vi "App - analyze RUS V6.vi"() -> ()   [LabVIEW 2015] (continued)
"z (pi/2)"=0.44352845258494766+0.2180214777125745i, "z center"=0.028000000000000025+0.0040000000000000036i, "z(0)"=-0.18602147771257446+0.41952845258494764i, "radius"=0.4674067691314655}}, "timestamp(min)"=396.73333333432674, "timestamp"=timestamp(3493751625 s since 1904-01-01), "Magn Field(T)"=0.0}, {"temperature"=137.004, "lorentzian"={"Amplitude"=0.00024818777938784227, "omega(0)"=668.2077960895239, "Gamma"=0.053536500417424936, "phase"=3.575640217162926, "Q"=12481.349936575929, "Norm  Ampl"=0.024927732275848467, "z (inf)"=0.22381537528742693-0.41844465648109325i, "4corners"={"z (-pi/2)"=-0.3944446564810932-0.1918153752874269i, "z(inf)"=0.22381537528742693-0.41844465648109325i, "z (pi/2)"=0.4504446564810933+0.1998153752874269i, "z center"=0.028000000000000025+0.0040000000000000036i, "z(0)"=-0.16781537528742688+0.42644465648109325i, "radius"=0.46562125057645803}}, "timestamp(min)"=398.0666666701436, "timestamp"=timestamp(3493751705 s since 1904-01-01), "Magn Field(T)"=0.0}, {"temperature"=136.689, "lorentzian"={"Amplitude"=0.0002522590875798226, "omega(0)"=668.216668111389, "Gamma"=0.053803366985016095, "phase"=3.6082228025377545, "Q"=12419.606904851944, "Norm  Ampl"=0.02511881590690244, "z (inf)"=0.23803210631804037-0.4129506304339384i, "4corners"={"z (-pi/2)"=-0.3889506304339384-0.20603210631804034i, "z(inf)"=0.23803210631804037-0.4129506304339384i, "z (pi/2)"=0.44495063043393845+0.21403210631804034i, "z center"=0.028000000000000025+0.0040000000000000036i, "z(0)"=-0.18203210631804032+0.42095063043393843i, "radius"=0.46686327110156284}}, "timestamp(min)"=399.3833333328366, "timestamp"=timestamp(3493751784 s since 1904-01-01), "Magn Field(T)"=0.0}, {"temperature"=136.379, "lorentzian"={"Amplitude"=0.0002437959945548481, "omega(0)"=668.2220891882298, "Gamma"=0.052047760738563105, "phase"=3.5758353326684773, "Q"=12838.632819281545, "Norm  Ampl"=0.0242465841922333, "z (inf)"=0.22399512738349894-0.4186163112320136i, "4corners"={"z (-pi/2)"=-0.3946163112320136-0.19199512738349891i, "z(inf)"=0.22399512738349894-0.4186163112320136i, "z (pi/2)"=0.4506163112320136+0.19999512738349892i, "z center"=0.028000000000000025+0.0040000000000000036i, "z(0)"=-0.1679951273834989+0.4266163112320136i, "radius"=0.4658525909313247}}, "timestamp(min)"=400.7166666686535, "timestamp"=timestamp(3493751864 s since 1904-01-01), "Magn Field(T)"=0.0}, {"temperature"=136.08, "lorentzian"={"Amplitude"=0.00024364628649236486, "omega(0)"=668.2279899714331, "Gamma"=0.05257683433154817, "phase"=3.562128551223608, "Q"=12709.551620350601, "Norm  Ampl"=0.02452040469231934, "z (inf)"=0.2183965576468025-0.4217378607902434i, "4corners"={"z (-pi/2)"=-0.39773786079024337-0.18639655764680246i, "z(inf)"=0.2183965576468025-0.4217378607902434i, "z (pi/2)"=0.4537378607902434+0.19439655764680247i, "z center"=0.028000000000000025+0.0040000000000000036i, "z(0)"=-0.16239655764680244+0.4297378607902434i, "radius"=0.4663727857347648}}, "timestamp(min)"=402.0333333313465, "timestamp"=timestamp(3493751943 s since 1904-01-01), "Magn Field(T)"=0.0}, {"temperature"=135.77, "lorentzian"={"Amplitude"=0.00022800803606069718, "omega(0)"=668.2341074013727, "Gamma"=0.049576251679184384, "phase"=3.5174097869555605, "Q"=13478.91550425432, "Norm  Ampl"=0.023118481798097362, "z (inf)"=0.19915533730309165-0.42977618112069815i, "4corners"={"z (-pi/2)"=-0.40577618112069813-0.16715533730309162i, "z(inf)"=0.19915533730309165-0.42977618112069815i, "z (pi/2)"=0.4617761811206982+0.17515533730309163i, "z center"=0.028000000000000025+0.0040000000000000036i, "z(0)"=-0.1431553373030916+0.43777618112069816i, "radius"=0.4663216966805124}}, "timestamp(min)"=403.3500000014901, "timestamp"=timestamp(3493752022 s since 1904-01-01), "Magn Field(T)"=0.0}, {"temperature"=135.475, "lorentzian"={"Amplitude"=0.00021967242445661102, "omega(0)"=668.2403250081744, "Gamma"=0.048208626694876563, "phase"=3.5063922887652854, "Q"=13861.426280354768, "Norm  Ampl"=0.02254989139105604, "z (inf)"=0.19487774885740458-0.43297576868681537i, "4corners"={"z (-pi/2)"=-0.40897576868681534-0.16287774885740455i, "z(inf)"=0.19487774885740458-0.43297576868681537i, "z (pi/2)"=0.4649757686868154+0.17087774885740456i, "z center"=0.028000000000000025+0.0040000000000000036i, "z(0)"=-0.13887774885740453+0.4409757686868154i, "radius"=0.4677563526913858}}, "timestamp(min)"=404.683333337307, "timestamp"=timestamp(3493752102 s since 1904-01-01), "Magn Field(T)"=0.0}, {"temperature"=135.167, "lorentzian"={"Amplitude"=0.00022045956380851477, "omega(0)"=668.2467222103966, "Gamma"=0.04866848493880481, "phase"=3.5042890577355816, "Q"=13730.584032986486, "Norm  Ampl"=0.022778847947626805, "z (inf)"=0.19405932289046807-0.4335919440676238i, "4corners"={"z (-pi/2)"=-0.4095919440676238-0.16205932289046804i, "z(inf)"=0.19405932289046807-0.4335919440676238i, "z (pi/2)"=0.46559194406762383+0.17005932289046805i, "z center"=0.028000000000000025+0.0040000000000000036i, "z(0)"=-0.13805932289046802+0.4415919440676238i, "radius"=0.4680410326368011}}, "timestamp(min)"=406.0, "timestamp"=timestamp(3493752181 s since 1904-01-01), "Magn Field(T)"=0.0}, {"temperature"=134.859, "lorentzian"={"Amplitude"=0.00020373450011305496, "omega(0)"=668.2497252249998, "Gamma"=0.04534069328819745, "phase"=3.4590588773416715, "Q"=14738.409952786287, "Norm  Ampl"=0.021363968760541766, "z (inf)"=0.1750860858123121-0.4436420009483996i, "4corners"={"z (-pi/2)"=-0.4196420009483996-0.14308608581231208i, "z(inf)"=0.1750860858123121-0.4436420009483996i, "z (pi/2)"=0.47564200094839965+0.1510860858123121i, "z center"=0.028000000000000025+0.0040000000000000036i, "z(0)"=-0.11908608581231206+0.4516420009483996i, "radius"=0.471187518566307}}, "timestamp(min)"=407.3166666701436, "timestamp"=timestamp(3493752260 s since 1904-01-01), "Magn Field(T)"=0.0}, {"temperature"=134.565, "lorentzian"={"Amplitude"=0.00022308585172458564, "omega(0)"=668.2550593154574, "Gamma"=0.04913914581717594, "phase"=3.50838853037322, "Q"=13599.240446745365, "Norm  Ampl"=0.02307832843849415, "z (inf)"=0.20442977527987274-0.43441189720743484i, "4corners"={"z (-pi/2)"=-0.4024118972074348-0.1644297752798727i, "z(inf)"=0.20442977527987274-0.43441189720743484i, "z (pi/2)"=0.4744118972074349+0.17242977527987272i, "z center"=0.03600000000000003+0.0040000000000000036i, "z(0)"=-0.13242977527987268+0.44241189720743485i, "radius"=0.46965261716916984}}, "timestamp(min)"=408.6499999985099, "timestamp"=timestamp(3493752340 s since 1904-01-01), "Magn Field(T)"=0.0}, {"temperature"=134.259, "lorentzian"={"Amplitude"=0.000209359984950497, "omega(0)"=668.2609151074342, "Gamma"=0.04650212304347896, "phase"=3.5133547690153906, "Q"=14370.546361563273, "Norm  Ampl"=0.02182407268942164, "z (inf)"=0.19848174926920006-0.4332540514538913i, "4corners"={"z (-pi/2)"=-0.40925405145389127-0.16648174926920004i, "z(inf)"=0.19848174926920006-0.4332540514538913i, "z (pi/2)"=0.4652540514538913+0.17448174926920004i, "z center"=0.028000000000000025+0.0040000000000000036i, "z(0)"=-0.14248174926920001+0.4412540514538913i, "radius"=0.4693134691725016}}, "timestamp(min)"=409.9666666686535, "timestamp"=timestamp(3493752419 s since 1904-01-01), "Magn Field(T)"=0.0}, {"temperature"=133.967, "lorentzian"={"Amplitude"=0.00016795569051138588, "omega(0)"=668.2619254491482, "Gamma"=0.04198266024418475, "phase"=3.3789707396391027, "Q"=15917.56981483118, "Norm  Ampl"=0.017415878698290484, "z (inf)"=0.14155055450548604-0.31120218603325117i, "4corners"={"z (-pi/2)"=-0.3592021860332511-0.005550554505486041i, "z(inf)"=0.14155055450548604-0.31120218603325117i, "z (pi/2)"=0.4472021860332512+0.18955055450548597i, "z center"=0.04400000000000004+0.09199999999999997i, "z(0)"=-0.05355055450548597+0.4952021860332511i, "radius"=0.4148350437298183}}, "timestamp(min)"=411.30000000447035, "timestamp"=timestamp(3493752499 s since 1904-01-01), "Magn Field(T)"=0.0}, {"temperature"=133.655, "lorentzian"={"Amplitude"=0.00020618932515028255, "omega(0)"=668.270115071191, "Gamma"=0.046136883483514225, "phase"=3.5346323148739778, "Q"=14484.509238903822, "Norm  Ampl"=0.021552558999279797, "z (inf)"=0.20691517073138083-0.42752368430412885i, "4corners"={"z (-pi/2)"=-0.4035236843041288-0.1749151707313808i, "z(inf)"=0.20691517073138083-0.42752368430412885i, "z (pi/2)"=0.4595236843041289+0.1829151707313808i, "z center"=0.028000000000000025+0.0040000000000000036i, "z(0)"=-0.15091517073138078+0.43552368430412886i, "radius"=0.4671437984531622}}, "timestamp(min)"=412.6166666671634, "timestamp"=timestamp(3493752578 s since 1904-01-01), "Magn Field(T)"=0.0}, {"temperature"=133.359, "lorentzian"={"Amplitude"=0.00019301381489978157, "omega(0)"=668.276245083583, "Gamma"=0.04348621694234654, "phase"=3.531368153146456, "Q"=15367.5415355071, "Norm  Ampl"=0.02015177614748303, "z (inf)"=0.20408538557141195-0.4246479987406104i, "4corners"={"z (-pi/2)"=-0.40064799874061036-0.17208538557141193i, "z(inf)"=0.20408538557141195-0.4246479987406104i, "z (pi/2)"=0.4566479987406104+0.18008538557141193i, "z center"=0.028000000000000025+0.0040000000000000036i, "z(0)"=-0.1480853855714119+0.4326479987406104i, "radius"=0.4634060528695791}}, "timestamp(min)"=413.933333337307, "timestamp"=timestamp(3493752657 s since 1904-01-01), "Magn Field(T)"=0.0}, {"temperature"=133.076, "lorentzian"={"Amplitude"=0.00019974392460320753, "omega(0)"=668.2795802722522, "Gamma"=0.04461745326656678, "phase"=3.53671447289831, "Q"=14977.985773406179, "Norm  Ampl"=0.020699137011803485, "z (inf)"=0.21457417147702626-0.4241791203195198i, "4corners"={"z (-pi/2)"=-0.3921791203195198-0.17457417147702622i, "z(inf)"=0.21457417147702626-0.4241791203195198i, "z (pi/2)"=0.46417912031951986+0.18257417147702623i, "z center"=0.03600000000000003+0.0040000000000000036i, "z(0)"=-0.1425741714770262+0.4321791203195198i, "radius"=0.46392466392325404}}, "timestamp(min)"=415.26666666567326, "timestamp"=timestamp(3493752737 s since 1904-01-01), "Magn Field(T)"=0.0}, {"temperature"=132.767, "lorentzian"={"Amplitude"=0.00020954228159723317, "omega(0)"=668.2870233031718, "Gamma"=0.046821008502632336, "phase"=3.6004118876433644, "Q"=14273.230002416542, "Norm  Ampl"=0.021889480609721925, "z (inf)"=0.24305720211583082-0.41516193523764255i, "4corners"={"z (-pi/2)"=-0.3831619352376425-0.20305720211583078i, "z(inf)"=0.24305720211583082-0.41516193523764255i, "z (pi/2)"=0.4551619352376426+0.2110572021158308i, "z center"=0.03600000000000003+0.0040000000000000036i, "z(0)"=-0.17105720211583075+0.42316193523764256i, "radius"=0.46751407775616943}}, "timestamp(min)"=416.58333333581686, "timestamp"=timestamp(3493752816 s since 1904-01-01), "Magn Field(T)"=0.0}, {"temperature"=132.465, "lorentzian"={"Amplitude"=0.00019413049707023668, "omega(0)"=668.2869168107318, "Gamma"=0.04319877501840161, "phase"=3.55325340676782, "Q"=15470.043225208541, "Norm  Ampl"=0.020176299526293698, "z (inf)"=0.2148844854302435-0.42403811821360354i, "4corners"={"z (-pi/2)"=-0.4000381182136035-0.18288448543024347i, "z(inf)"=0.2148844854302435-0.42403811821360354i, "z (pi/2)"=0.45603811821360357+0.19088448543024347i, "z center"=0.028000000000000025+0.0040000000000000036i, "z(0)"=-0.15888448543024344+0.43203811821360355i, "radius"=0.46705721441636006}}, "timestamp(min)"=417.91666666418314, "timestamp"=timestamp(3493752896 s since 1904-01-01), "Magn Field(T)"=0.0}, {"temperature"=132.185, "lorentzian"={"Amplitude"=0.00020122225797151018, "omega(0)"=668.2934784041765, "Gamma"=0.04497947268960905, "phase"=3.5446976448663943, "Q"=14857.74373158809, "Norm  Ampl"=0.020912876525446128, "z (inf)"=0.21038601556727435-0.4316763214619255i, "4corners"={"z (-pi/2)"=-0.3996763214619255-0.18638601556727433i, "z(inf)"=0.21038601556727435-0.4316763214619255i, "z (pi/2)"=0.45567632146192555+0.17838601556727432i, "z center"=0.028000000000000025-0.0040000000000000036i, "z(0)"=-0.1543860155672743+0.4236763214619255i, "radius"=0.4649426788473073}}, "timestamp(min)"=419.23333333432674, "timestamp"=timestamp(3493752975 s since 1904-01-01), "Magn Field(T)"=0.0}, {"temperature"=131.882, "lorentzian"={"Amplitude"=0.00017903490059702695, "omega(0)"=668.3008315870534, "Gamma"=0.04055671373632796, "phase"=3.5607932411011722, "Q"=16478.180059949846, "Norm  Ampl"=0.018542520405159534, "z (inf)"=0.21409420197942536-0.41361295774797074i, "4corners"={"z (-pi/2)"=-0.3896129577479707-0.18209420197942533i, "z(inf)"=0.21409420197942536-0.41361295774797074i, "z (pi/2)"=0.4456129577479708+0.19009420197942534i, "z center"=0.028000000000000025+0.0040000000000000036i, "z(0)"=-0.1580942019794253+0.42161295774797075i, "radius"=0.45719977525078415}}, "timestamp(min)"=420.55000000447035, "timestamp"=timestamp(3493753054 s since 1904-01-01), "Magn Field(T)"=0.0}, {"temperature"=131.592, "lorentzian"={"Amplitude"=0.00017776941850395074, "omega(0)"=668.3028814309054, "Gamma"=0.040071528004769166, "phase"=3.556601894504015, "Q"=16677.748883231165, "Norm  Ampl"=0.018550360511525102, "z (inf)"=0.21465311273870263-0.419634170792521i, "4corners"={"z (-pi/2)"=-0.395634170792521-0.1826531127387026i, "z(inf)"=0.21465311273870263-0.419634170792521i, "z (pi/2)"=0.45163417079252105+0.1906531127387026i, "z center"=0.028000000000000025+0.0040000000000000036i, "z(0)"=-0.15865311273870258+0.42763417079252103i, "radius"=0.4629311991625902}}, "timestamp(min)"=421.8833333328366, "timestamp"=timestamp(3493753134 s since 1904-01-01), "Magn Field(T)"=0.0}, {"temperature"=131.299, "lorentzian"={"Amplitude"=0.00013151959831981622, "omega(0)"=668.3062964998082, "Gamma"=0.03348268101980571, "phase"=3.467971571661652, "Q"=19959.760573070325, "Norm  Ampl"=0.01370925850354954, "z (inf)"=0.17527374281445499-0.29582856805960495i, "4corners"={"z (-pi/2)"=-0.3438285680596049-0.039273742814454976i, "z(inf)"=0.17527374281445499-0.29582856805960495i, "z (pi/2)"=0.43182856805960496+0.22327374281445492i, "z center"=0.04400000000000004+0.09199999999999997i, "z(0)"=-0.08727374281445491+0.4798285680596049i, "radius"=0.40944327293982896}}, "timestamp(min)"=423.20000000298023, "timestamp"=timestamp(3493753213 s since 1904-01-01), "Magn Field(T)"=0.0}, {"temperature"=131.007, "lorentzian"={"Amplitude"=0.00014024604190308675, "omega(0)"=668.3103990781085, "Gamma"=0.0354379197218754, "phase"=3.487085072823789, "Q"=18858.623878691407, "Norm  Ampl"=0.014555488747515302, "z (inf)"=0.183098526053321-0.29446138419265844i, "4corners"={"z (-pi/2)"=-0.34246138419265837-0.04709852605332099i, "z(inf)"=0.183098526053321-0.29446138419265844i, "z (pi/2)"=0.43046138419265845+0.23109852605332093i, "z center"=0.04400000000000004+0.09199999999999997i, "z(0)"=-0.09509852605332092+0.4784613841926584i, "radius"=0.4107320311618171}}, "timestamp(min)"=424.51666666567326, "timestamp"=timestamp(3493753292 s since 1904-01-01), "Magn Field(T)"=0.0}, {"temperature"=130.718, "lorentzian"={"Amplitude"=0.00018728871691243128, "omega(0)"=668.310674127471, "Gamma"=0.04173713236217242, "phase"=3.4962997673810627, "Q"=16012.37642126991, "Norm  Ampl"=0.019142027382721867, "z (inf)"=0.18729046326062257-0.43408232050414974i, "4corners"={"z (-pi/2)"=-0.4020823205041497-0.16329046326062255i, "z(inf)"=0.18729046326062257-0.43408232050414974i, "z (pi/2)"=0.45808232050414976+0.15529046326062254i, "z center"=0.028000000000000025-0.0040000000000000036i, "z(0)"=-0.13129046326062252+0.42608232050414974i, "radius"=0.4586330276986361}}, "timestamp(min)"=425.8500000014901, "timestamp"=timestamp(3493753372 s since 1904-01-01), "Magn Field(T)"=0.0}, {"temperature"=130.427, "lorentzian"={"Amplitude"=0.00013102976571802591, "omega(0)"=668.3160212015783, "Gamma"=0.03289666447607903, "phase"=3.479634497746158, "Q"=20315.616547919246, "Norm  Ampl"=0.013442055183748003, "z (inf)"=0.18751308439089182-0.293489351771138i, "4corners"={"z (-pi/2)"=-0.3334893517711379-0.0435130843908918i, "z(inf)"=0.18751308439089182-0.293489351771138i, "z (pi/2)"=0.437489351771138+0.22751308439089174i, "z center"=0.052000000000000046+0.09199999999999997i, "z(0)"=-0.08351308439089172+0.47748935177113794i, "radius"=0.40861453274457227}}, "timestamp(min)"=427.16666666418314, "timestamp"=timestamp(3493753451 s since 1904-01-01), "Magn Field(T)"=0.0}, {"temperature"=130.147, "lorentzian"={"Amplitude"=0.00019806996039286532, "omega(0)"=668.3205621538442, "Gamma"=0.04395504205226639, "phase"=3.5868870379071494, "Q"=15204.639353072454, "Norm  Ampl"=0.02022729371515346, "z (inf)"=0.22621098732741798-0.4193063264724261i, "4corners"={"z (-pi/2)"=-0.3873063264724261-0.20221098732741796i, "z(inf)"=0.22621098732741798-0.4193063264724261i, "z (pi/2)"=0.4433063264724261+0.19421098732741796i, "z center"=0.028000000000000025-0.0040000000000000036i, "z(0)"=-0.17021098732741793+0.4113063264724261i, "radius"=0.46018142107796056}}, "timestamp(min)"=428.5, "timestamp"=timestamp(3493753531 s since 1904-01-01), "Magn Field(T)"=0.0}, {"temperature"=129.849, "lorentzian"={"Amplitude"=0.00018012359308280804, "omega(0)"=668.3261810591241, "Gamma"=0.03572807603918743, "phase"=3.617601804019526, "Q"=18705.910173447, "Norm  Ampl"=0.01846804924972829, "z (inf)"=0.17686465617028402-0.4314417557280484i, "4corners"={"z (-pi/2)"=-0.5194417557280484-0.208864656170284i, "z(inf)"=0.17686465617028402-0.4314417557280484i, "z (pi/2)"=0.3994417557280484+0.26486465617028404i, "z center"=-0.06+0.028000000000000025i, "z(0)"=-0.296864656170284+0.48744175572804843i, "radius"=0.5169057866276393}}, "timestamp(min)"=429.8166666701436, "timestamp"=timestamp(3493753610 s since 1904-01-01), "Magn Field(T)"=0.0}, {"temperature"=129.561, "lorentzian"={"Amplitude"=0.0002515206474333576, "omega(0)"=668.3339307703254, "Gamma"=0.05293578222265151, "phase"=3.697878467065015, "Q"=12625.371775168398, "Norm  Ampl"=0.026109156013374792, "z (inf)"=0.24843944779595978-0.5028560864052527i, "4corners"={"z (-pi/2)"=-0.43085608640525264-0.3444394477959598i, "z(inf)"=0.24843944779595978-0.5028560864052527i, "z (pi/2)"=0.4068560864052526+0.17643944779595977i, "z center"=-0.01200000000000001-0.08400000000000002i, "z(0)"=-0.2724394477959598+0.3348560864052526i, "radius"=0.4932232020971732}}, "timestamp(min)"=431.1333333328366, "timestamp"=timestamp(3493753689 s since 1904-01-01), "Magn Field(T)"=0.0}, {"temperature"=129.282, "lorentzian"={"Amplitude"=0.00019009529834722127, "omega(0)"=668.3324079597492, "Gamma"=0.042712971939908764, "phase"=3.5856365991332066, "Q"=15647.059373438127, "Norm  Ampl"=0.019869211365660003, "z (inf)"=0.2278387908458529-0.42406748951978035i, "4corners"={"z (-pi/2)"=-0.3920674895197803-0.20383879084585288i, "z(inf)"=0.2278387908458529-0.42406748951978035i, "z (pi/2)"=0.44806748951978037+0.19583879084585287i, "z center"=0.028000000000000025-0.0040000000000000036i, "z(0)"=-0.17183879084585285+0.41606748951978034i, "radius"=0.465179791132615}}, "timestamp(min)"=432.4666666686535, "timestamp"=timestamp(3493753769 s since 1904-01-01), "Magn Field(T)"=0.0}, {"temperature"=128.991, "lorentzian"={"Amplitude"=0.00020743270166107407, "omega(0)"=668.3322615543187, "Gamma"=0.04692462104458906, "phase"=3.5328468712785126, "Q"=14242.677866684338, "Norm  Ampl"=0.021731792084702495, "z (inf)"=0.2046104571630927-0.4321239265355797i, "4corners"={"z (-pi/2)"=-0.40012392653557965-0.18061045716309268i, "z(inf)"=0.2046104571630927-0.4321239265355797i, "z (pi/2)"=0.4561239265355797+0.17261045716309267i, "z center"=0.028000000000000025-0.0040000000000000036i, "z(0)"=-0.14861045716309265+0.4241239265355797i, "radius"=0.4631213124566813}}, "timestamp(min)"=433.7833333313465, "timestamp"=timestamp(3493753848 s since 1904-01-01), "Magn Field(T)"=0.0}, {"temperature"=128.717, "lorentzian"={"Amplitude"=0.00014057972242425618, "omega(0)"=668.3288000801537, "Gamma"=0.0350239817019726, "phase"=3.350369108098308, "Q"=19082.03372669397, "Norm  Ampl"=0.014440672605235712, "z (inf)"=0.12945625364420338-0.3113549647555858i, "4corners"={"z (-pi/2)"=-0.3593549647555857+0.006543746355796645i, "z(inf)"=0.12945625364420338-0.3113549647555858i, "z (pi/2)"=0.4473549647555858+0.1774562536442033i, "z center"=0.04400000000000004+0.09199999999999997i, "z(0)"=-0.041456253644203286+0.4953549647555857i, "radius"=0.41230813584003195}}, "timestamp(min)"=435.1000000014901, "timestamp"=timestamp(3493753927 s since 1904-01-01), "Magn Field(T)"=0.0}, {"temperature"=128.421, "lorentzian"={"Amplitude"=0.00018912094504794594, "omega(0)"=668.3337947654519, "Gamma"=0.0420370819340677, "phase"=3.45940499769483, "Q"=15898.672410556183, "Norm  Ampl"=0.019525044126968823, "z (inf)"=0.18114246269768364-0.44521177378260157i, "4corners"={"z (-pi/2)"=-0.40521177378260154-0.1491424626976836i, "z(inf)"=0.18114246269768364-0.44521177378260157i, "z (pi/2)"=0.4772117737826016+0.1411424626976836i, "z center"=0.03600000000000003-0.0040000000000000036i, "z(0)"=-0.10914246269768357+0.43721177378260156i, "radius"=0.46447191928289705}}, "timestamp(min)"=436.433333337307, "timestamp"=timestamp(3493754007 s since 1904-01-01), "Magn Field(T)"=0.0}, {"temperature"=128.135, "lorentzian"={"Amplitude"=0.0001945195497852276, "omega(0)"=668.3393724178951, "Gamma"=0.043849594993256275, "phase"=3.4896884528609635, "Q"=15241.631593648253, "Norm  Ampl"=0.020523623085199085, "z (inf)"=0.18765440283338847-0.44397435687764764i, "4corners"={"z (-pi/2)"=-0.4119743568776476-0.16365440283338845i, "z(inf)"=0.18765440283338847-0.44397435687764764i, "z (pi/2)"=0.46797435687764766+0.15565440283338844i, "z center"=0.028000000000000025-0.0040000000000000036i, "z(0)"=-0.13165440283338842+0.43597435687764763i, "radius"=0.46804589844798933}}, "timestamp(min)"=437.75, "timestamp"=timestamp(3493754086 s since 1904-01-01), "Magn Field(T)"=0.0}, {"temperature"=127.874, "lorentzian"={"Amplitude"=0.000190466492974867, "omega(0)"=668.3408415336296, "Gamma"=0.04304683332538277, "phase"=3.5244127391147786, "Q"=15525.900278930372, "Norm  Ampl"=0.02009953162829439, "z (inf)"=0.2104132227577419-0.43712420258490553i, "4corners"={"z (-pi/2)"=-0.3971242025849055-0.17841322275774188i, "z(inf)"=0.2104132227577419-0.43712420258490553i, "z (pi/2)"=0.46912420258490556+0.17041322275774187i, "z center"=0.03600000000000003-0.0040000000000000036i, "z(0)"=-0.13841322275774184+0.4291242025849055i, "radius"=0.4669224208983244}}, "timestamp(min)"=439.08333333581686, "timestamp"=timestamp(3493754166 s since 1904-01-01), "Magn Field(T)"=0.0}, {"temperature"=127.58, "lorentzian"={"Amplitude"=0.00017614434719281864, "omega(0)"=668.3350781624661, "Gamma"=0.03977774583620109, "phase"=3.4103259526571854, "Q"=16801.733333873963, "Norm  Ampl"=0.018474740713941437, "z (inf)"=0.15131608902790966-0.45177914883439746i, "4corners"={"z (-pi/2)"=-0.41977914883439743-0.12731608902790964i, "z(inf)"=0.15131608902790966-0.45177914883439746i, "z (pi/2)"=0.4757791488343975+0.11931608902790963i, "z center"=0.028000000000000025-0.0040000000000000036i, "z(0)"=-0.09531608902790961+0.44377914883439745i, "radius"=0.4644491618508928}}, "timestamp(min)"=440.3999999985099, "timestamp"=timestamp(3493754245 s since 1904-01-01), "Magn Field(T)"=0.0}, {"temperature"=127.303, "lorentzian"={"Amplitude"=0.000178448287164071, "omega(0)"=668.341978511539, "Gamma"=0.04075165439042157, "phase"=3.458727986906405, "Q"=16400.36431670928, "Norm  Ampl"=0.018933127124076275, "z (inf)"=0.18088296555633987-0.44542949587281366i, "4corners"={"z (-pi/2)"=-0.40542949587281363-0.14888296555633984i, "z(inf)"=0.18088296555633987-0.44542949587281366i, "z (pi/2)"=0.4774294958728137+0.14088296555633983i, "z center"=0.03600000000000003-0.0040000000000000036i, "z(0)"=-0.1088829655563398+0.43742949587281366i, "radius"=0.4645977545521781}}, "timestamp(min)"=441.7166666686535, "timestamp"=timestamp(3493754324 s since 1904-01-01), "Magn Field(T)"=0.0}, {"temperature"=127.032, "lorentzian"={"Amplitude"=0.0001793737910586766, "omega(0)"=668.3443633787955, "Gamma"=0.04031506960918336, "phase"=3.482825666306089, "Q"=16578.028262328822, "Norm  Ampl"=0.018801002983454388, "z (inf)"=0.19206426889851805-0.43546318642137727i, "4corners"={"z (-pi/2)"=-0.40346318642137724-0.152064268898518i, "z(inf)"=0.19206426889851805-0.43546318642137727i, "z (pi/2)"=0.4754631864213773+0.16006426889851802i, "z center"=0.03600000000000003+0.0040000000000000036i, "z(0)"=-0.12006426889851798+0.4434631864213773i, "radius"=0.46635174305073546}}, "timestamp(min)"=443.05000000447035, "timestamp"=timestamp(3493754404 s since 1904-01-01), "Magn Field(T)"=0.0}, {"temperature"=126.745, "lorentzian"={"Amplitude"=0.00017473128234191018, "omega(0)"=668.3397547361191, "Gamma"=0.03922736347643625, "phase"=3.4158312259381005, "Q"=17037.59048546784, "Norm  Ampl"=0.018213770062324868, "z (inf)"=0.16174244705836888-0.45096228744718125i, "4corners"={"z (-pi/2)"=-0.4109622874471812-0.12974244705836885i, "z(inf)"=0.16174244705836888-0.45096228744718125i, "z (pi/2)"=0.4829622874471813+0.12174244705836884i, "z center"=0.03600000000000003-0.0040000000000000036i, "z(0)"=-0.08974244705836881+0.44296228744718125i, "radius"=0.46431287877060157}}, "timestamp(min)"=444.3666666671634, "timestamp"=timestamp(3493754483 s since 1904-01-01), "Magn Field(T)"=0.0}, {"temperature"=126.472, "lorentzian"={"Amplitude"=0.00016985229184637778, "omega(0)"=668.338634717693, "Gamma"=0.038548010622264324, "phase"=3.36580870245142, "Q"=17337.824285325845, "Norm  Ampl"=0.017944948936428617, "z (inf)"=0.1395051514979586-0.4578694336986776i, "4corners"={"z (-pi/2)"=-0.4178694336986776-0.1075051514979586i, "z(inf)"=0.1395051514979586-0.4578694336986776i, "z (pi/2)"=0.48986943369867764+0.09950515149795859i, "z center"=0.03600000000000003-0.0040000000000000036i, "z(0)"=-0.06750515149795856+0.4498694336986776i, "radius"=0.46552205021091503}}, "timestamp(min)"=445.70000000298023, "timestamp"=timestamp(3493754563 s since 1904-01-01), "Magn Field(T)"=0.0}, {"temperature"=126.195, "lorentzian"={"Amplitude"=0.0001697476143014984, "omega(0)"=668.3411059711797, "Gamma"=0.0389192723855822, "phase"=3.400885738644188, "Q"=17172.49745446858, "Norm  Ampl"=0.0181237265906366, "z (inf)"=0.15539779092559663-0.45410803111628234i, "4corners"={"z (-pi/2)"=-0.4141080311162823-0.12339779092559659i, "z(inf)"=0.15539779092559663-0.45410803111628234i, "z (pi/2)"=0.48610803111628237+0.11539779092559659i, "z center"=0.03600000000000003-0.0040000000000000036i, "z(0)"=-0.08339779092559656+0.44610803111628233i, "radius"=0.46567485669003933}}, "timestamp(min)"=447.01666666567326, "timestamp"=timestamp(3493754642 s since 1904-01-01), "Magn Field(T)"=0.0}, {"temperature"=125.926, "lorentzian"={"Amplitude"=0.00014967332960728232, "omega(0)"=668.3387712789065, "Gamma"=0.03405009771839295, "phase"=3.343347027084076, "Q"=19628.10141710365, "Norm  Ampl"=0.015778792659266735, "z (inf)"=0.1288598639328376-0.4579999888655082i, "4corners"={"z (-pi/2)"=-0.41799998886550815-0.09685986393283756i, "z(inf)"=0.1288598639328376-0.4579999888655082i, "z (pi/2)"=0.4899999888655082+0.08885986393283755i, "z center"=0.03600000000000003-0.0040000000000000036i, "z(0)"=-0.056859863932837526+0.4499999888655082i, "radius"=0.4633993355837993}}, "timestamp(min)"=448.33333333581686, "timestamp"=timestamp(3493754721 s since 1904-01-01), "Magn Field(T)"=0.0}, {"temperature"=125.648, "lorentzian"={"Amplitude"=0.00015890027273297025, "omega(0)"=668.3427557708224, "Gamma"=0.03654471251520353, "phase"=3.4071524057178104, "Q"=18288.35718690562, "Norm  Ampl"=0.017102639047579412, "z (inf)"=0.15882428088801925-0.45558704635195746i, "4corners"={"z (-pi/2)"=-0.4155870463519574-0.12682428088801923i, "z(inf)"=0.15882428088801925-0.45558704635195746i, "z (pi/2)"=0.4875870463519575+0.1188242808880192i, "z center"=0.03600000000000003-0.0040000000000000036i, "z(0)"=-0.08682428088801918+0.44758704635195745i, "radius"=0.46799216276401895}}, "timestamp(min)"=449.66666666418314, "timestamp"=timestamp(3493754801 s since 1904-01-01), "Magn Field(T)"=0.0}, {"temperature"=125.371, "lorentzian"={"Amplitude"=0.00014113258135423898, "omega(0)"=668.3438270287197, "Gamma"=0.0328359775535354, "phase"=3.4224417889228933, "Q"=20354.010351574263, "Norm  Ampl"=0.015317995908975795, "z (inf)"=0.16530066288420467-0.4442230921647853i, "4corners"={"z (-pi/2)"=-0.41222309216478525-0.12530066288420463i, "z(inf)"=0.16530066288420467-0.4442230921647853i, "z (pi/2)"=0.4842230921647853+0.13330066288420464i, "z center"=0.03600000000000003+0.0040000000000000036i, "z(0)"=-0.0933006628842046+0.4522230921647853i, "radius"=0.4665003770331342}}, "timestamp(min)"=450.98333333432674, "timestamp"=timestamp(3493754880 s since 1904-01-01), "Magn Field(T)"=0.0}, {"temperature"=125.102, "lorentzian"={"Amplitude"=0.0001429072723984059, "omega(0)"=668.3463481103089, "Gamma"=0.03319261106950844, "phase"=3.4922376591079947, "Q"=20135.395396003318, "Norm  Ampl"=0.015660205089643275, "z (inf)"=0.19806430364890984-0.439089658276503i, "4corners"={"z (-pi/2)"=-0.40708965827650295-0.1580643036489098i, "z(inf)"=0.19806430364890984-0.439089658276503i, "z (pi/2)"=0.479089658276503+0.1660643036489098i, "z center"=0.03600000000000003+0.0040000000000000036i, "z(0)"=-0.12606430364890978+0.447089658276503i, "radius"=0.47179792685936445}}, "timestamp(min)"=452.30000000447035, "timestamp"=timestamp(3493754959 s since 1904-01-01), "Magn Field(T)"=0.0}, {"temperature"=124.83, "lorentzian"={"Amplitude"=0.00013813052592595213, "omega(0)"=668.3455084349229, "Gamma"=0.03220463241618305, "phase"=3.4504535565686507, "Q"=20753.08607152661, "Norm  Ampl"=0.015278154630597103, "z (inf)"=0.18020770874129619-0.4479597969299136i, "4corners"={"z (-pi/2)"=-0.4159597969299136-0.14020770874129615i, "z(inf)"=0.18020770874129619-0.4479597969299136i, "z (pi/2)"=0.48795979692991365+0.14820770874129616i, "z center"=0.03600000000000003+0.0040000000000000036i, "z(0)"=-0.10820770874129612+0.4559597969299136i, "radius"=0.474408601630855}}, "timestamp(min)"=453.6333333328366, "timestamp"=timestamp(3493755039 s since 1904-01-01), "Magn Field(T)"=0.0}, {"temperature"=124.565, "lorentzian"={"Amplitude"=0.0001241550689128081, "omega(0)"=668.3450708618282, "Gamma"=0.029302305447045547, "phase"=3.3705378321996333, "Q"=22808.61729701255, "Norm  Ampl"=0.013845225294181049, "z (inf)"=0.1432331585027775-0.4561669504399603i, "4corners"={"z (-pi/2)"=-0.4241669504399603-0.10323315850277746i, "z(inf)"=0.1432331585027775-0.4561669504399603i, "z (pi/2)"=0.49616695043996034+0.11123315850277747i, "z center"=0.03600000000000003+0.0040000000000000036i, "z(0)"=-0.07123315850277744+0.4641669504399603i, "radius"=0.47249610851275237}}, "timestamp(min)"=454.95000000298023, "timestamp"=timestamp(3493755118 s since 1904-01-01), "Magn Field(T)"=0.0}, {"temperature"=124.29, "lorentzian"={"Amplitude"=0.00013600574422085066, "omega(0)"=668.3433267141062, "Gamma"=0.03222809761528601, "phase"=3.303602764581753, "Q"=20737.90810404851, "Norm  Ampl"=0.015235315667254033, "z (inf)"=0.11225308169717747-0.4625435119875039i, "4corners"={"z (-pi/2)"=-0.43054351198750385-0.07225308169717744i, "z(inf)"=0.11225308169717747-0.4625435119875039i, "z (pi/2)"=0.5025435119875039+0.08025308169717744i, "z center"=0.03600000000000003+0.0040000000000000036i, "z(0)"=-0.04025308169717741+0.4705435119875039i, "radius"=0.4727339431920989}}, "timestamp(min)"=456.2833333313465, "timestamp"=timestamp(3493755198 s since 1904-01-01), "Magn Field(T)"=0.0}, {"temperature"=124.019, "lorentzian"={"Amplitude"=0.00011823441411221721, "omega(0)"=668.3444873126522, "Gamma"=0.027985877204057336, "phase"=3.332408594972943, "Q"=23881.491455117117, "Norm  Ampl"=0.013390117286503522, "z (inf)"=0.13474472920756247-0.46577566662945014i, "4corners"={"z (-pi/2)"=-0.4257756666294501-0.08674472920756245i, "z(inf)"=0.13474472920756247-0.46577566662945014i, "z (pi/2)"=0.5137756666294502+0.09474472920756245i, "z center"=0.04400000000000004+0.0040000000000000036i, "z(0)"=-0.04674472920756241+0.47377566662945014i, "radius"=0.4784598027380128}}, "timestamp(min)"=457.6000000014901, "timestamp"=timestamp(3493755277 s since 1904-01-01), "Magn Field(T)"=0.0}, {"temperature"=123.76, "lorentzian"={"Amplitude"=0.00010252866822353009, "omega(0)"=668.3461478794261, "Gamma"=0.02452701411914777, "phase"=3.382096592555638, "Q"=27249.388964866335, "Norm  Ampl"=0.011669477357501797, "z (inf)"=0.14932717477975163-0.45008670777708876i, "4corners"={"z (-pi/2)"=-0.42608670777708874-0.10132717477975159i, "z(inf)"=0.14932717477975163-0.45008670777708876i, "z (pi/2)"=0.4980867077770888+0.1253271747797516i, "z center"=0.03600000000000003+0.01200000000000001i, "z(0)"=-0.07732717477975157+0.4740867077770888i, "radius"=0.4757805944422586}}, "timestamp(min)"=458.91666666418314, "timestamp"=timestamp(3493755356 s since 1904-01-01), "Magn Field(T)"=0.0}, {"temperature"=123.485, "lorentzian"={"Amplitude"=0.00010060670392465627, "omega(0)"=668.3457969116931, "Gamma"=0.023856627563744223, "phase"=3.3710756033915925, "Q"=28015.099582952047, "Norm  Ampl"=0.011503947995463478, "z (inf)"=0.15369068173587727-0.46557023087952365i, "4corners"={"z (-pi/2)"=-0.4255702308795236-0.10569068173587723i, "z(inf)"=0.15369068173587727-0.46557023087952365i, "z (pi/2)"=0.5135702308795237+0.11369068173587724i, "z center"=0.04400000000000004+0.0040000000000000036i, "z(0)"=-0.0656906817358772+0.47357023087952366i, "radius"=0.48221182833681164}}, "timestamp(min)"=460.25, "timestamp"=timestamp(3493755436 s since 1904-01-01), "Magn Field(T)"=0.0}, {"temperature"=123.221, "lorentzian"={"Amplitude"=6.834880513297458e-05, "omega(0)"=668.3464465453555, "Gamma"=0.014499364014175118, "phase"=3.348175852611088, "Q"=46094.8801541885, "Norm  Ampl"=0.00790720989531802, "z (inf)"=0.051860271604710725-0.48175324618211113i, "4corners"={"z (-pi/2)"=-0.5937532461821111-0.05986027160471068i, "z(inf)"=0.051860271604710725-0.48175324618211113i, "z (pi/2)"=0.4737532461821112+0.16386027160471078i, "z center"=-0.06+0.052000000000000046i, "z(0)"=-0.17186027160471073+0.5857532461821112i, "radius"=0.5453487399576725}}, "timestamp(min)"=461.5666666701436, "timestamp"=timestamp(3493755515 s since 1904-01-01), "Magn Field(T)"=0.0}, {"temperature"=122.957, "lorentzian"={"Amplitude"=7.492110052105228e-05, "omega(0)"=668.3409387012916, "Gamma"=0.018251290582365107, "phase"=3.0627075354221365, "Q"=36618.83173056599, "Norm  Ampl"=0.008562087027053392, "z (inf)"=-0.0009683969973760531-0.46366339389332006i, "4corners"={"z (-pi/2)"=-0.43166339389332004+0.04096839699737609i, "z(inf)"=-0.0009683969973760531-0.46366339389332006i, "z (pi/2)"=0.5036633938933202-0.03296839699737608i, "z center"=0.03600000000000003+0.0040000000000000036i, "z(0)"=0.07296839699737612+0.47166339389332007i, "radius"=0.4691222786911471}}, "timestamp(min)"=462.8833333328366, "timestamp"=timestamp(3493755594 s since 1904-01-01), "Magn Field(T)"=0.0}, {"temperature"=122.69, "lorentzian"={"Amplitude"=5.654900216759101e-05, "omega(0)"=668.3392344820684, "Gamma"=0.014311546013530267, "phase"=3.002252756323969, "Q"=46699.303754480075, "Norm  Ampl"=0.006665806274545064, "z (inf)"=-0.036689733713346495-0.45724999789622234i, "4corners"={"z (-pi/2)"=-0.4332499978962223+0.06868973371334652i, "z(inf)"=-0.036689733713346495-0.45724999789622234i, "z (pi/2)"=0.48924999789622237-0.060689733713346516i, "z center"=0.028000000000000025+0.0040000000000000036i, "z(0)"=0.09268973371334654+0.46524999789622234i, "radius"=0.4657642345727812}}, "timestamp(min)"=464.2166666686535, "timestamp"=timestamp(3493755674 s since 1904-01-01), "Magn Field(T)"=0.0}, {"temperature"=122.431, "lorentzian"={"Amplitude"=5.253092552595975e-05, "omega(0)"=668.3394447248988, "Gamma"=0.013166746708605508, "phase"=3.0229439738552664, "Q"=50759.64925246768, "Norm  Ampl"=0.006259458515548345, "z (inf)"=-0.028273218082330583-0.46805672919298136i, "4corners"={"z (-pi/2)"=-0.44405672919298134+0.06027321808233061i, "z(inf)"=-0.028273218082330583-0.46805672919298136i, "z (pi/2)"=0.5000567291929814-0.052273218082330604i, "z center"=0.028000000000000025+0.0040000000000000036i, "z(0)"=0.08427321808233063+0.47605672919298136i, "radius"=0.47539902255864736}}, "timestamp(min)"=465.5333333313465, "timestamp"=timestamp(3493755753 s since 1904-01-01), "Magn Field(T)"=0.0}, {"temperature"=122.165, "lorentzian"={"Amplitude"=3.8069276236775707e-05, "omega(0)"=668.3369686011712, "Gamma"=0.00956916586627817, "phase"=2.740366878421992, "Q"=69842.7614214941, "Norm  Ampl"=0.004631131869139208, "z (inf)"=-0.15301072213580735-0.44152902070318667i, "4corners"={"z (-pi/2)"=-0.40952902070318664+0.1930107221358074i, "z(inf)"=-0.15301072213580735-0.44152902070318667i, "z (pi/2)"=0.4815290207031867-0.18501072213580738i, "z center"=0.03600000000000003+0.0040000000000000036i, "z(0)"=0.22501072213580742+0.4495290207031867i, "radius"=0.4839640083426039}}, "timestamp(min)"=466.8666666671634, "timestamp"=timestamp(3493755833 s since 1904-01-01), "Magn Field(T)"=0.0}, {"temperature"=121.901, "lorentzian"={"Amplitude"=3.7380373777561024e-05, "omega(0)"=668.3366293662327, "Gamma"=0.009524463760762934, "phase"=2.785011252220867, "Q"=70170.52572760246, "Norm  Ampl"=0.004567471078013794, "z (inf)"=-0.13139835622846566-0.4453856374038484i, "4corners"={"z (-pi/2)"=-0.41338563740384837+0.1713983562284657i, "z(inf)"=-0.13139835622846566-0.4453856374038484i, "z (pi/2)"=0.48538563740384844-0.16339835622846569i, "z center"=0.03600000000000003+0.0040000000000000036i, "z(0)"=0.20339835622846572+0.4533856374038484i, "radius"=0.479551520457245}}, "timestamp(min)"=468.183333337307, "timestamp"=timestamp(3493755912 s since 1904-01-01), "Magn Field(T)"=0.0}, {"temperature"=121.649, "lorentzian"={"Amplitude"=4.835511572480418e-05, "omega(0)"=668.3323623372692, "Gamma"=0.012039669526169004, "phase"=2.751412986430426, "Q"=55510.85608160634, "Norm  Ampl"=0.006033634076691258, "z (inf)"=-0.1466132372572539-0.4674803785525046i, "4corners"={"z (-pi/2)"=-0.4194803785525046+0.18661323725725393i, "z(inf)"=-0.1466132372572539-0.4674803785525046i, "z (pi/2)"=0.5074803785525046-0.19461323725725393i, "z center"=0.04400000000000004-0.0040000000000000036i, "z(0)"=0.23461323725725397+0.4594803785525046i, "radius"=0.5011461538522103}}, "timestamp(min)"=469.5, "timestamp"=timestamp(3493755991 s since 1904-01-01), "Magn Field(T)"=0.0}, {"temperature"=121.386, "lorentzian"={"Amplitude"=4.840869092525542e-05, "omega(0)"=668.3318352391343, "Gamma"=0.012235175401509526, "phase"=2.7648855248135082, "Q"=54623.804997244115, "Norm  Ampl"=0.0058895434900639075, "z (inf)"=-0.14107391096360036-0.44360899316941477i, "4corners"={"z (-pi/2)"=-0.41160899316941474+0.1810739109636004i, "z(inf)"=-0.14107391096360036-0.44360899316941477i, "z (pi/2)"=0.4836089931694148-0.1730739109636004i, "z center"=0.03600000000000003+0.0040000000000000036i, "z(0)"=0.21307391096360043+0.4516089931694148i, "radius"=0.48136159039757453}}, "timestamp(min)"=470.83333333581686, "timestamp"=timestamp(3493756071 s since 1904-01-01), "Magn Field(T)"=0.0}, {"temperature"=121.132, "lorentzian"={"Amplitude"=7.347521340555284e-05, "omega(0)"=668.3346922322422, "Gamma"=0.017628843913302102, "phase"=3.306656500176045, "Q"=37911.4305804217, "Norm  Ampl"=0.008601569674681083, "z (inf)"=0.116173696891024-0.47729395393669627i, "4corners"={"z (-pi/2)"=-0.44529395393669624-0.07617369689102396i, "z(inf)"=0.116173696891024-0.47729395393669627i, "z (pi/2)"=0.5172939539366963+0.08417369689102397i, "z center"=0.03600000000000003+0.0040000000000000036i, "z(0)"=-0.044173696891023934+0.4852939539366963i, "radius"=0.487925908073339}}, "timestamp(min)"=472.1499999985099, "timestamp"=timestamp(3493756150 s since 1904-01-01), "Magn Field(T)"=0.0}, {"temperature"=120.874, "lorentzian"={"Amplitude"=5.6673592067554466e-05, "omega(0)"=668.3330864941908, "Gamma"=0.013354810010371709, "phase"=3.4296317238697673, "Q"=50044.3724751715, "Norm  Ampl"=0.006660960287860126, "z (inf)"=0.1776865152020266-0.4742207412003794i, "4corners"={"z (-pi/2)"=-0.44222074120037935-0.13768651520202657i, "z(inf)"=0.1776865152020266-0.4742207412003794i, "z (pi/2)"=0.5142207412003794+0.14568651520202658i, "z center"=0.03600000000000003+0.0040000000000000036i, "z(0)"=-0.10568651520202654+0.4822207412003794i, "radius"=0.49876862963134955}}, "timestamp(min)"=473.48333333432674, "timestamp"=timestamp(3493756230 
